vi "PS Configure Power Supply Source Settings.vi"(0 "DAQmx Task In":refnum<k21>, 5 "Channel Settings":T1={"Voltage Setpoint(V)"=0.0, "Current Setpoint(A)"=0.0, "Remote Sense"=16095, "Idle Output Behavior"=12528, "Enable Output?"=FALSE} {"Idle Output Behavior" items=["Disable output when Task stopped"=15503, "Maintain Existing Value"=12528]; "Remote Sense" items=["Local"=16095, "Remote"=16096]; "Voltage Setpoint(V)" format="%#.2p"; "Current Setpoint(A)" format="%#.2p"}, 11 "error in (no error)":errorcluster) -> (4 "DAQmx Task Out":refnum<k21>, 15 "error out":errorcluster)   [LabVIEW 2021, in "DAQ_Power Supply Source and Measure.lvlib"]
doc: "Configure channel settings needed for the power supply source task"
uses:
  DAQ_Power Supply Source and Measure.lvlib
  Typedefs/Channel Settings.ctl
  <resource>/objmgr/daqmx.rc
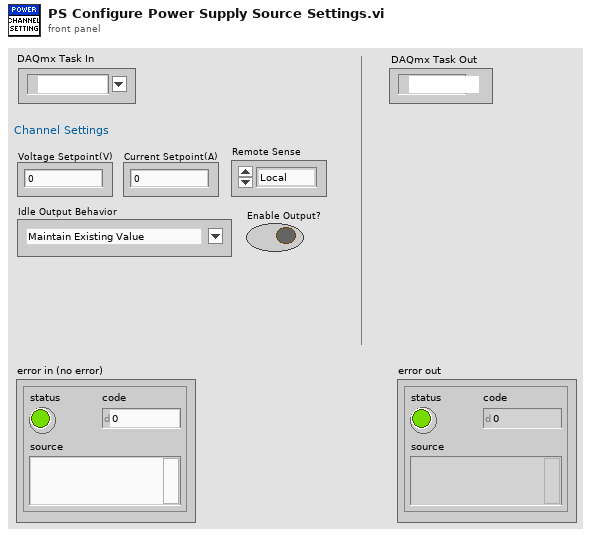
[diagram p1: front panel]
types:
  T1 = typedef "DAQ_Power Supply Source and Measure.lvlib/Channel Settings.ctl" = cluster{"Voltage Setpoint(V)":dbl, "Current Setpoint(A)":dbl, "Remote Sense":i32, "Idle Output Behavior":i32, "Enable Output?":bool}
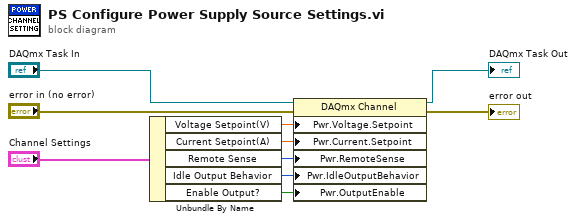
[diagram p0: block diagram]
diagram:
  n1 = Unbundle By Name("Channel Settings") -> ("Voltage Setpoint(V)"=w1:dbl, "Current Setpoint(A)"=w2:dbl, "Remote Sense"=w3:i32, "Idle Output Behavior"=w4:i32, "Enable Output?"=w5:bool)
  n2 = property class="DAQmx Channel"(reference="DAQmx Task In", error in="error in (no error)", "Pwr.Voltage.Setpoint"=w1, "Pwr.Current.Setpoint"=w2, "Pwr.RemoteSense"=w3, "Pwr.IdleOutputBehavior"=w4, "Pwr.OutputEnable"=w5) -> (reference out=→"DAQmx Task Out":refnum<k21>, error out=→"error out":errorcluster)
